vi "MISC Comment White Space.vi"(11 "Input String":string) -> (3 "Output String":string)   [LabVIEW 2017]
doc: "This routine performs a find and replace on each element pair in the search and replace arrays. The elements in search and replace arrays are fixed to operate on all white space characters."
panel:
  in  "Replace Text Array":string[](array[string])=["<CR>", "<LF>", "<T>"]
  in  "Search Text Array":string[](array[string])=["\r", "\n", "\t"]
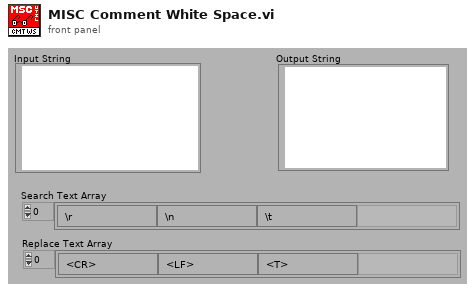
[diagram p1: front panel]
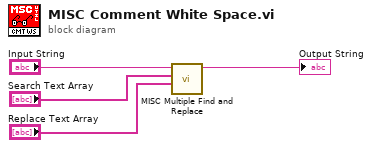
[diagram p0: block diagram]
diagram:
  n1 = call "MISC Multiple Find and Replace.vi"("Replace Text Array"="Replace Text Array", "Search Text Array"="Search Text Array", "Input String"="Input String") -> ("Output String"=→"Output String":string)  [unwired: 8 out]
